vi "Get All Status Refs.vi"(8 "error in (no error)":errorcluster, 10 "framework configuration in":T1, 11 "VeriStand Data Sharing Framework in":refnum<class "VeriStand DSF.lvclass">) -> (0 "error out":errorcluster, 1 "contiguous?":bool, 2 "all channel offsets":u64[](array[numeric]) format="%.0x", 3 "VeriStand Data Sharing Framework out":refnum<class "VeriStand DSF.lvclass">)   [LabVIEW 2017, in "DSF Engine.lvlib" / "VeriStand DSF.lvclass"]
uses:
  VeriStand DSF.lvclass
  DSF Core.lvlibp/Typedefs/DSF Engine Framework Configuration.ctl
  DSF Core.lvlibp/Typedefs/DSF Engine Plugin Configuration.ctl
  DSF Core.lvlibp/Typedefs/DSF Timing Info.ctl
  DSF Core.lvlibp/Typedefs/DSF Engine Plugin Thread Configuration.ctl
  DSF Core.lvlibp/Typedefs/DSF Settings Info.ctl
  DSF Core.lvlibp/Typedefs/DSF Engine Transfer Group Configuration.ctl
  DSF Core.lvlibp/Typedefs/DSF Direction.ctl
  DSF Core.lvlibp/Typedefs/DSF Engine Transfer Configuration.ctl
  DSF Core.lvlibp/Typedefs/DSF Byte Order.ctl
  DSF Core.lvlibp/Typedefs/DSF Engine Channel Configuration.ctl
  DSF Core.lvlibp/Typedefs/DSF Data Type.ctl
  DSF Core.lvlibp/Typedefs/DSF Timeout Behavior.ctl
  VeriStand DSF.lvclass/VeriStand DSF.ctl
  <vilib>/NI Veristand/Custom Device API/Data Access Type.ctl
  DSF Core.lvlibp/Classes/Configuration/Channel Count (Transfer).vi
  <vilib>/NI Veristand/Custom Device API/Custom Device API.lvlib
  DSF Core.lvlibp
  DSF Core.lvlibp/Classes/Configuration/Configuration Session.lvclass
  Shared/DSF Shared.lvlib
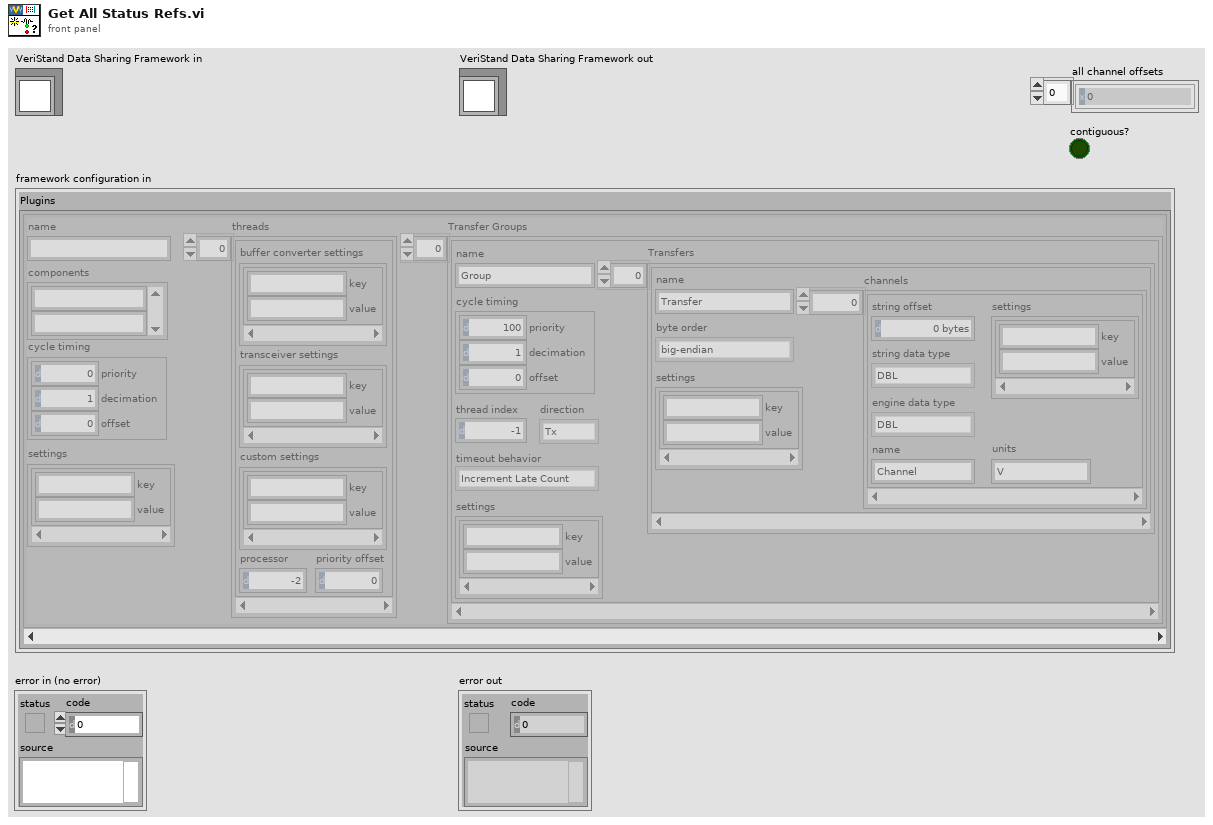
[diagram p1: front panel]
types:
  T1 = typedef "DSF Core.lvlibp/DSF Engine Framework Configuration.ctl" = cluster{"Plugins":T2[]}
  T2 = typedef "DSF Core.lvlibp/DSF Engine Plugin Configuration.ctl" = cluster{"name":string, "components":string[], "cycle timing":T3, "threads":T4[], "Transfer Groups":T6[], "settings":T5}
  T3 = typedef "DSF Core.lvlibp/DSF Timing Info.ctl" = cluster{"priority":u64, "decimation":u64, "offset":u64}
  T4 = typedef "DSF Core.lvlibp/DSF Engine Plugin Thread Configuration.ctl" = cluster{"buffer converter settings":T5, "transceiver settings":T5, "custom settings":T5, "processor":i32, "priority offset":i16}
  T5 = typedef "DSF Core.lvlibp/DSF Settings Info.ctl" = cluster{"key":string, "value":string}[]
  T6 = typedef "DSF Core.lvlibp/DSF Engine Transfer Group Configuration.ctl" = cluster{"name":string, "direction":T7, "cycle timing":T3, "thread index":i32, "settings":T5, "Transfers":T8[], "timeout behavior":T12}
  T7 = typedef "DSF Core.lvlibp/DSF Direction.ctl" = enum8{"Tx", "Rx"}
  T8 = typedef "DSF Core.lvlibp/DSF Engine Transfer Configuration.ctl" = cluster{"name":string, "byte order":T9, "settings":T5, "channels":T10[]}
  T9 = typedef "DSF Core.lvlibp/DSF Byte Order.ctl" = enum8{"big-endian", "little-endian"}
  T10 = typedef "DSF Core.lvlibp/DSF Engine Channel Configuration.ctl" = cluster{"string offset":u64, "string data type":T11, "engine data type":T11, "name":string, "settings":T5, "units":string}
  T11 = typedef "DSF Core.lvlibp/DSF Data Type.ctl" = enum8{"Bool", "SGL", "DBL", "I8", "I16", "I32", "I64", "U8", "U16", "U32", "U64"}
  T12 = typedef "DSF Core.lvlibp/DSF Timeout Behavior.ctl" = enum8{"Increment Late Count", "Throw Error"}
  T13 = typedef "Custom Device API.lvlib/Custom Device Item Ref.ctl" = u64
  T14 = typedef "Custom Device API.lvlib/Data Access Type.ctl" = enum16{"Read", "Write"}
  T15 = typedef "Custom Device API.lvlib/Data Reference.ctl" = i32
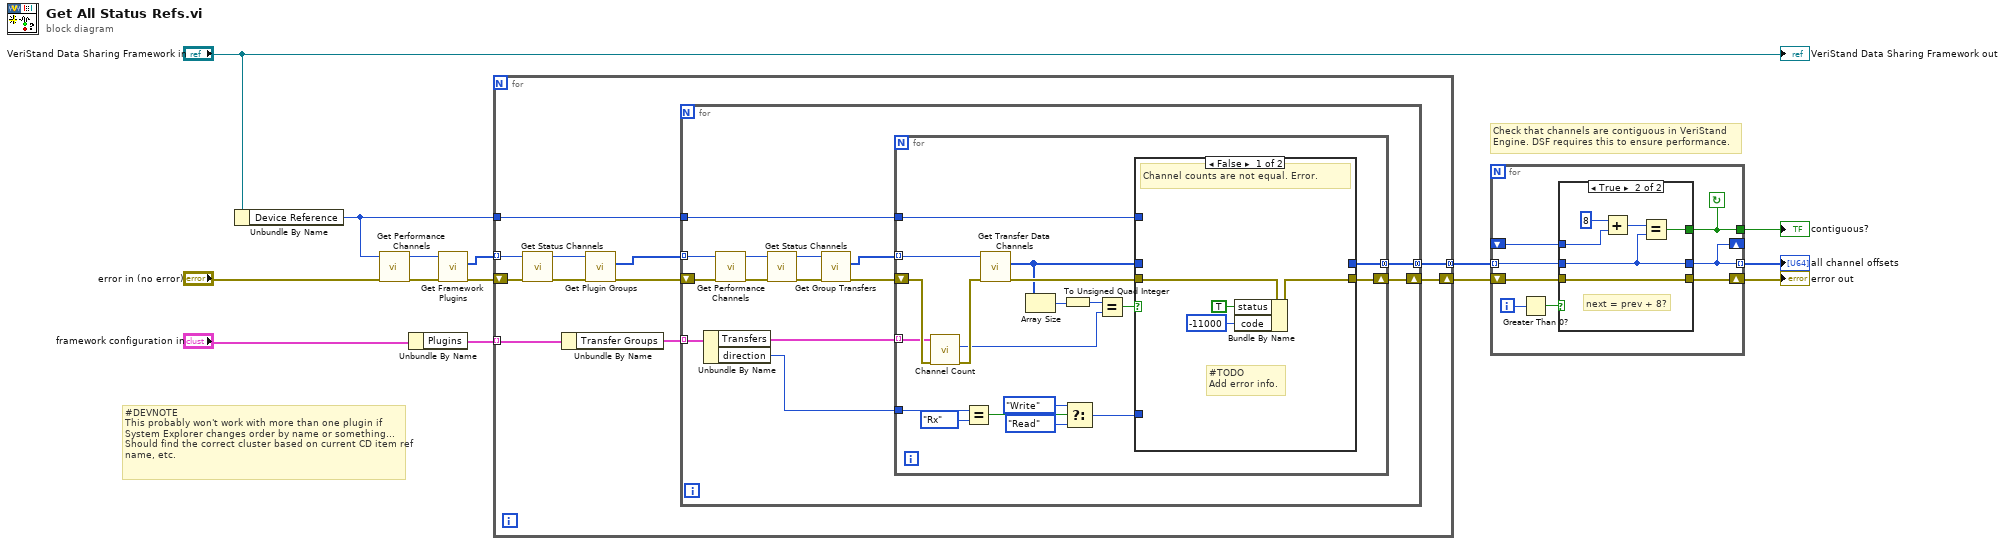
[diagram p0: block diagram]
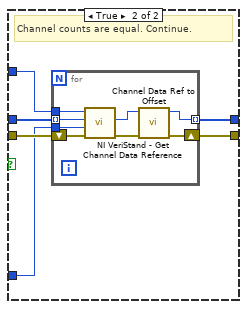
[diagram p2: hidden frame]
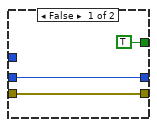
[diagram p3: hidden frame]
diagram:
  # "#DEVNOTE\nThis probably won't work with more than one plugin if System Explorer changes order by name or something... Should find the correct cluster based on current CD item ref name, etc."
  # "Check that channels are contiguous in VeriStand Engine. DSF requires this to ensure performance."
  n1 = Unbundle By Name("VeriStand Data Sharing Framework in") -> ("Device Reference"=w2:T13)
  n2 = call "Get Performance Channels.vi"("error in (no error)"="error in (no error)", "Item Ref in"=w2) -> ("error out"=w3:errorcluster, "Item Ref out"=w1:T13)  [unwired: 7 in, 1 out]
  n3 = Unbundle By Name("framework configuration in") -> ("Plugins"=w13:T2[])
  n4 = call "Get Framework Plugins.vi"("error in (no error)"=w3, "Framework Ref in"=w1) -> ("error out"=w6:errorcluster, "Plugin refs"=w5:T13[])  [unwired: 7 in, 1 out]
  n5 = for {
    tunnel: w5 -> [w18] mode=indexing
    tunnel: w13 -> [w25] mode=indexing
    tunnel: w2 -> [w24]
    shift-right: [w23] -> w11
    shift-left: w6 -> [w17]
    tunnel: [w22] -> w10 mode=concatenating
    n6 = call "Get Status Channels.vi"("error in (no error)"=w17, "Item Ref in"=w18) -> ("error out"=w16:errorcluster, "Item Ref out"=w15:T13)  [unwired: 7 in, 1 out]
    n7 = Unbundle By Name(w25) -> ("Transfer Groups"=w21:T6[])
    n8 = call "Get Plugin Groups.vi"("error in (no error)"=w16, "Plugin Ref in"=w15) -> ("error out"=w20:errorcluster, "Group refs"=w19:T13[])  [unwired: 7 in, 1 out]
    n9 = for {
      tunnel: w21 -> [w39] mode=indexing
      tunnel: w19 -> [w31] mode=indexing
      tunnel: w24 -> [w38]
      shift-right: [w37] -> w23
      shift-left: w20 -> [w30]
      tunnel: [w36] -> w22 mode=concatenating
      n10 = Unbundle By Name(w39) -> ("Transfers"=w35:T8[], "direction"=w34:T7)
      n11 = call "Get Performance Channels.vi"("error in (no error)"=w30, "Item Ref in"=w31) -> ("error out"=w29:errorcluster, "Item Ref out"=w28:T13)  [unwired: 7 in, 1 out]
      n12 = call "Get Status Channels.vi"("error in (no error)"=w29, "Item Ref in"=w28) -> ("error out"=w27:errorcluster, "Item Ref out"=w26:T13)  [unwired: 7 in, 1 out]
      n13 = call "Get Group Transfers.vi"("error in (no error)"=w27, "Group Ref in"=w26) -> ("error out"=w33:errorcluster, "Transfer refs"=w32:T13[])  [unwired: 7 in, 1 out]
      n14 = for {
        tunnel: w35 -> [w47] mode=indexing
        tunnel: w32 -> [w43] mode=indexing
        tunnel: w34 -> [w57]
        tunnel: w38 -> [w50]
        shift-right: [w46] -> w37
        shift-left: w33 -> [w48]
        tunnel: [w45] -> w36 mode=concatenating
        n15 = call-poly "Channel Count.vi"("error in (no error)"=w48, "Transfer Configuration in"=w47) -> ("error out"=w44:errorcluster, "total channel count"=w40:u64)  [unwired: 7 in, 1 out]
        n16 = Equal?(x=w57, y=DSF_Direction."Rx") -> (x = y?=w55:bool)
        n17 = call "Get Transfer Data Channels.vi"("error in (no error)"=w44, "Transfer Ref in"=w43) -> ("error out"=w42:errorcluster, "Channels refs"=w41:T13[])  [unwired: 7 in, 1 out]
        n18 = Array Size(array=w41) -> (size(s)=w58:i32)
        n19 = To Unsigned Quad Integer(1:w58) -> (0:w51:u64)
        n20 = Select(t=Data_Access_Type."Write" ("Access"), s=w55, f=Data_Access_Type."Read") -> (s? t:f=w49:T14)
        n21 = Equal?(x=w51, y=w40) -> (x = y?=w52:bool)
        n22 = case shown="False" w52 {
          tunnel: w41 -> [_ w65]
          tunnel: w50 -> [_ w67]
          tunnel: w49 -> [_ w66]
          tunnel: w42 -> [w62 w68]
          tunnel: [w61 w63] -> w46
          tunnel: [_ w64] -> w45
          frame False {
            # "#TODO\nAdd error info."
            # "Channel counts are not equal. Error."
            n23 = Bundle By Name(cluster=w62, "status"=TRUE, "code"=-11000) -> (w61:errorcluster)
          }
          frame True {
            # "Channel counts are equal. Continue."
            n24 = for {
              tunnel: w67 -> [w75]
              tunnel: w66 -> [w74]
              tunnel: w65 -> [w73] mode=indexing
              tunnel: [w69] -> w64 mode=indexing
              shift-right: [w70] -> w63
              shift-left: w68 -> [w76]
              n25 = call <vilib>:"NI VeriStand - Get Channel Data Reference.vi"("error in (no error)"=w76, "Access"=w74, "Channel Ref in"=w73, "Device Ref in"=w75) -> ("error out"=w72:errorcluster, "Channel Data Reference"=w71:T15)  [unwired: 5 in, 1 out]
              n26 = call "Channel Data Ref to Offset.vi"("error in (no error)"=w72, "Channel Data Reference"=w71) -> ("error out"=w70:errorcluster, "channel offset"=w69:u64)  [unwired: 8 in]
            }
          }
        }
      }
    }
  }
  n27 = for {
    tunnel: w10 -> [w82] mode=indexing
    shift-right: [w79] -> w9
    shift-left: w11 -> [w81]
    shift-right: [w77] -> _
    shift-left: _ -> [w80]
    tunnel: [w78] -> w8
    tunnel: [w77] -> w7 mode=indexing
    i -> [w84]
    stop <- w78 continue-if-true
    n28 = Greater Than 0?(x=w84) -> (x > 0?=w83:bool)
    n29 = case shown="True" w83 {
      tunnel: w82 -> [w86 w89]
      tunnel: w81 -> [w87 w88]
      tunnel: w80 -> [_ w93]
      tunnel: [w87 w88] -> w79
      tunnel: [TRUE w90] -> w78
      tunnel: [w86 w89] -> w77
      frame False {
      }
      frame True {
        # "next = prev + 8?"
        n30 = Add(x=u64 8 ("y"), y=w93) -> (x+y=w91:u64)
        n31 = Equal?(x=w91, y=w89) -> (x = y?=w90:bool)
      }
    }
  }
  "error out" <- w9
  "all channel offsets" <- w7
  "contiguous?" <- w8
  "VeriStand Data Sharing Framework out" <- "VeriStand Data Sharing Framework in"
